vi "z物镜移动.vi"(7 "停止":bool, 8 "position":dbl, 9 "maxVelocity":dbl=5.0, 10 "SerialNumber":string="27000001", 11 "KCubeDCServoControl":refnum<k24>(container)) -> (1 "当前位置":dbl, 2 "IsConnected":bool, 3 "CreateDevice":bool)   [LabVIEW 2015]
uses:
  C:/Users/Hongq/Documents/GitHub/TPP-3D-printer/Kinesis/Thorlabs.MotionControl.Controls.dll
  Kinesis/Thorlabs.MotionControl.Controls.dll
  C:/Users/Hongq/Documents/GitHub/TPP-3D-printer/Kinesis/ThorLabs.MotionControl.KCube.DCServoCLI.dll
  Kinesis/ThorLabs.MotionControl.KCube.DCServoCLI.dll
panel:
  out "错误输出":errorcluster={"status"=TRUE, "code"=1172, "source"="z物镜移动.vi中的调用节点 Error calling method Thorlabs.MotionControl.Controls.KCubeDCServoControl.CreateDevice, (System.Exception: BuildDeviceList failed with error code 7) <append><b>System.Exception</b>"}
  out "错误输出 2":errorcluster={"status"=TRUE, "code"=1172, "source"="z物镜移动.vi中的调用节点 Error calling method Thorlabs.MotionControl.KCube.DCServoCLI.KCubeDCServo.SetVelocityParams, (System.ArgumentNullException: 键不能为 null。\r\n参数名: key) <append><b>System.ArgumentNullException</b>"} caption="错误输出"
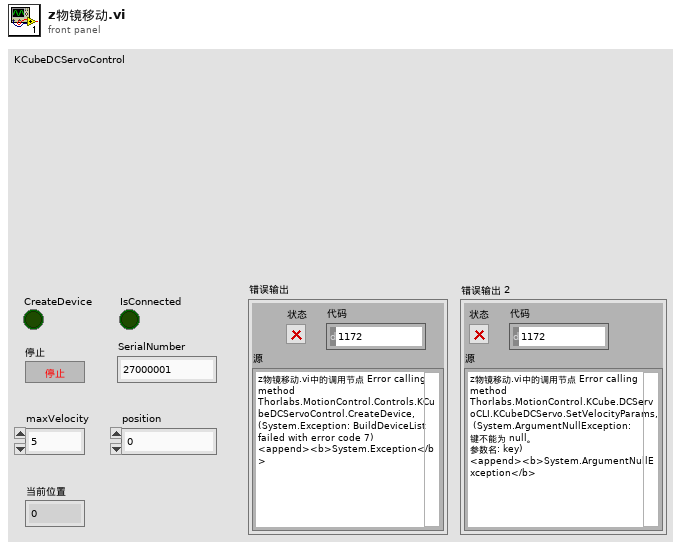
[diagram p1: front panel]
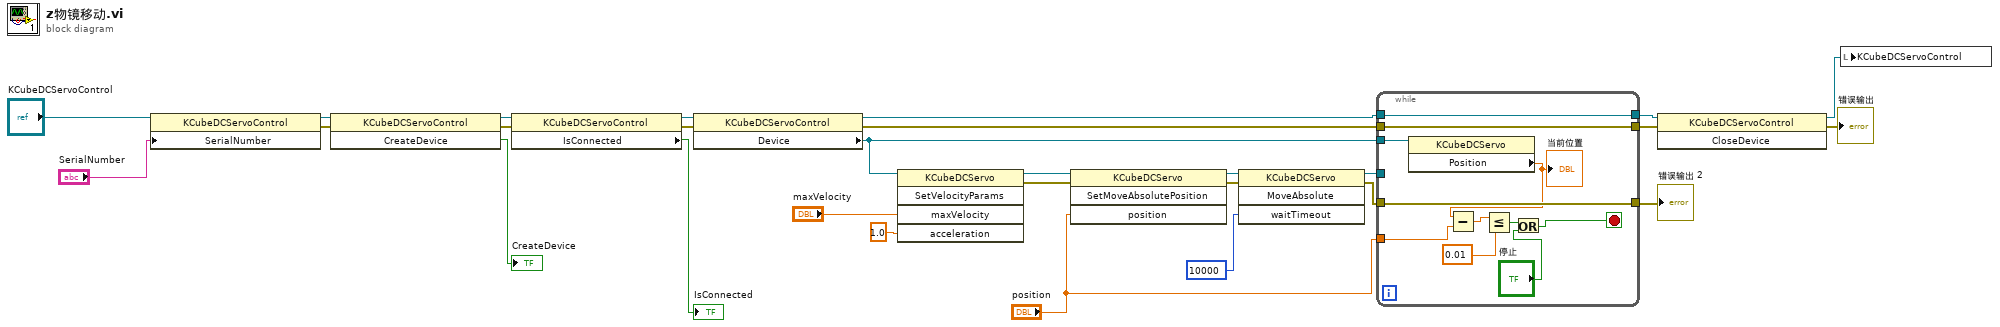
[diagram p0: block diagram]
diagram:
  n1 = property class="KCubeDCServoControl"(reference="KCubeDCServoControl", "SerialNumber"="SerialNumber") -> (reference out=w26:refnum<k24>, error out=w25:errorcluster)  [unwired: 1 in]
  n2 = invoke class="KCubeDCServoControl" method="CreateDevice"(reference=w26, error in=w25) -> (reference out=w19:refnum<k24>, error out=w17:errorcluster, "CreateDevice"=→"CreateDevice":bool)  [unwired: 1 in]
  n3 = property class="KCubeDCServoControl"(reference=w19, error in=w17) -> (reference out=w18:refnum<k24>, error out=w16:errorcluster, "IsConnected"=→"IsConnected":bool)
  n4 = property class="KCubeDCServoControl"(reference=w18, error in=w16) -> (reference out=w24:refnum<k24>, error out=w22:errorcluster, "Device"=w3:refnum<k24>)
  n5 = invoke class="KCubeDCServo" method="SetVelocityParams"(reference=w3, "maxVelocity"="maxVelocity", "acceleration"=1.0) -> (reference out=w12:refnum<k24>, error out=w11:errorcluster)  [unwired: 2 in, 3 out]
  n6 = invoke class="KCubeDCServo" method="SetMoveAbsolutePosition"(reference=w12, error in=w11, "position"="position") -> (reference out=w10:refnum<k24>, error out=w9:errorcluster)  [unwired: 1 in, 2 out]
  n7 = invoke class="KCubeDCServo" method="MoveAbsolute"(reference=w10, error in=w9, "waitTimeout"=10000) -> (reference out=w6:refnum<k24>, error out=w5:errorcluster)  [unwired: 1 in, 2 out]
  n8 = while {
    tunnel: [w39] -> w23
    tunnel: w24 -> [w39]
    tunnel: [w38] -> w21
    tunnel: w22 -> [w38]
    tunnel: w6 -> [_]
    tunnel: w5 -> [w36]
    tunnel: [w36] -> w4
    tunnel: w3 -> [w37]
    tunnel: "position" -> [w31]
    stop <- w33 stop-if-true
    n9 = property class="KCubeDCServo"(reference=w37) -> ("Position"=w32:dbl)  [unwired: 1 in, 2 out]
    "当前位置" <- w32
    n10 = Subtract(x=w32, y=w31) -> (x-y=w30:dbl)
    n11 = Less Or Equal?(x=w30, y=0.01) -> (x <= y?=w35:bool)
    n12 = Or(x=w35, y="停止") -> (x .or. y?=w33:bool)
  }
  "错误输出 2" <- w4
  n13 = invoke class="KCubeDCServoControl" method="CloseDevice"(reference=w23, error in=w21) -> (reference out=w1:refnum<k24>, error out=→"错误输出":errorcluster)  [unwired: 1 in, 1 out]
  n14 = local write "KCubeDCServoControl"(w1) -> ()
